vi "Teleop.vi"(10 "Match Info":T1={"Autonomous Elapsed Seconds"=0.0, "TeleOp Elapsed Seconds"=0.0, "Disabled Elapsed Seconds"=0.0, "Visited Autonomous"=FALSE, "Visited TeleOp"=FALSE, "Visited Disabled"=FALSE, "Autonomous Settings"={"Autonomous Style"=enum."Independent", "VI Refnum"=refnum}}, 11 "Call Context":T2) -> ()   [LabVIEW 2023]
doc: "This VI is called for each TeleOp packet received from the DS where the robot is not disabled. It is often used to read from the joysticks and update I/O or to update setpoints for timed control loops. It should complete and return within 20 milliseconds or it may miss DS packets."
uses:
  <vilib>/Rock Robotics/WPI/DriverStation/WPI_DriverStationDerivedRobotMode.ctl
  <vilib>/Rock Robotics/WPI/DriverStation/WPI_DriverStationMatch Info.ctl
  <vilib>/Rock Robotics/WPI/Utilities/WPI_GetSetVariantRefNum.vi
  <vilib>/Rock Robotics/Network Tables/NT Write Boolean Array.vi
  <vilib>/Rock Robotics/Network Tables/NT Write Numeric Array.vi
  <vilib>/Rock Robotics/Network Tables/NT Read Boolean.vi
  <vilib>/Rock Robotics/Network Tables/NT Read Number.vi
  <vilib>/Rock Robotics/WPI/ThirdParty/Phoenix-LabVIEW/Pigeon IMU/CTRE_PigeonIMU_GetYPR.vi
  <vilib>/Rock Robotics/Network Tables/NT Write Float.vi
panel:
  out "Yaw":dbl(knob) scale=-180.0..180.0
  out "Sample Slider 0":dbl(slide) scale=0.0..5.0
  out "Sample Boolean 1":bool
  out "Sample Boolean 0":bool
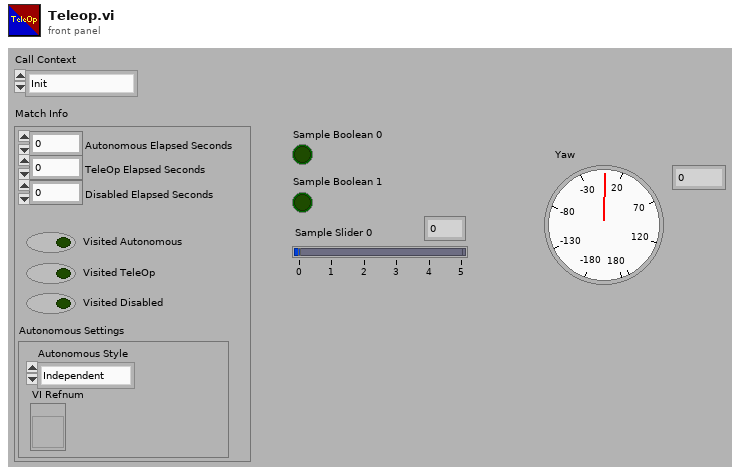
[diagram p1: front panel]
types:
  T1 = typedef "WPI_DriverStationMatch Info.ctl" = cluster{"Autonomous Elapsed Seconds":dbl, "TeleOp Elapsed Seconds":dbl, "Disabled Elapsed Seconds":dbl, "Visited Autonomous":bool, "Visited TeleOp":bool, "Visited Disabled":bool, "Autonomous Settings":cluster{"Autonomous Style":enum16{"Iterative", "Independent"}, "VI Refnum":refnum<vi>}}
  T2 = typedef "WPI_DriverStationDerivedRobotMode.ctl" = enum16{"Init", "Execute", "Stop"}
  T3 = typedef "WPI_JoystickDevRef.ctl" = cluster{"Device":T4}
  T4 = typedef "WPI_JoystickDeviceEnum.ctl" = enum16{"USB 0", "USB 1", "USB 2", "USB 3", "USB 4", "USB 5"}
  T5 = typedef "CTRE_PigeonIMU_DeviceRef.ctl" = cluster{"DeviceStatus":errorcluster, "Device Number":u8, "Type":T6, "Device ID":u32, "Handle":u64, "UsageFrame":u32, "Library Path":path}
  T6 = typedef "CTRE_PigeonIMU_ConnectionType.ctl" = u32
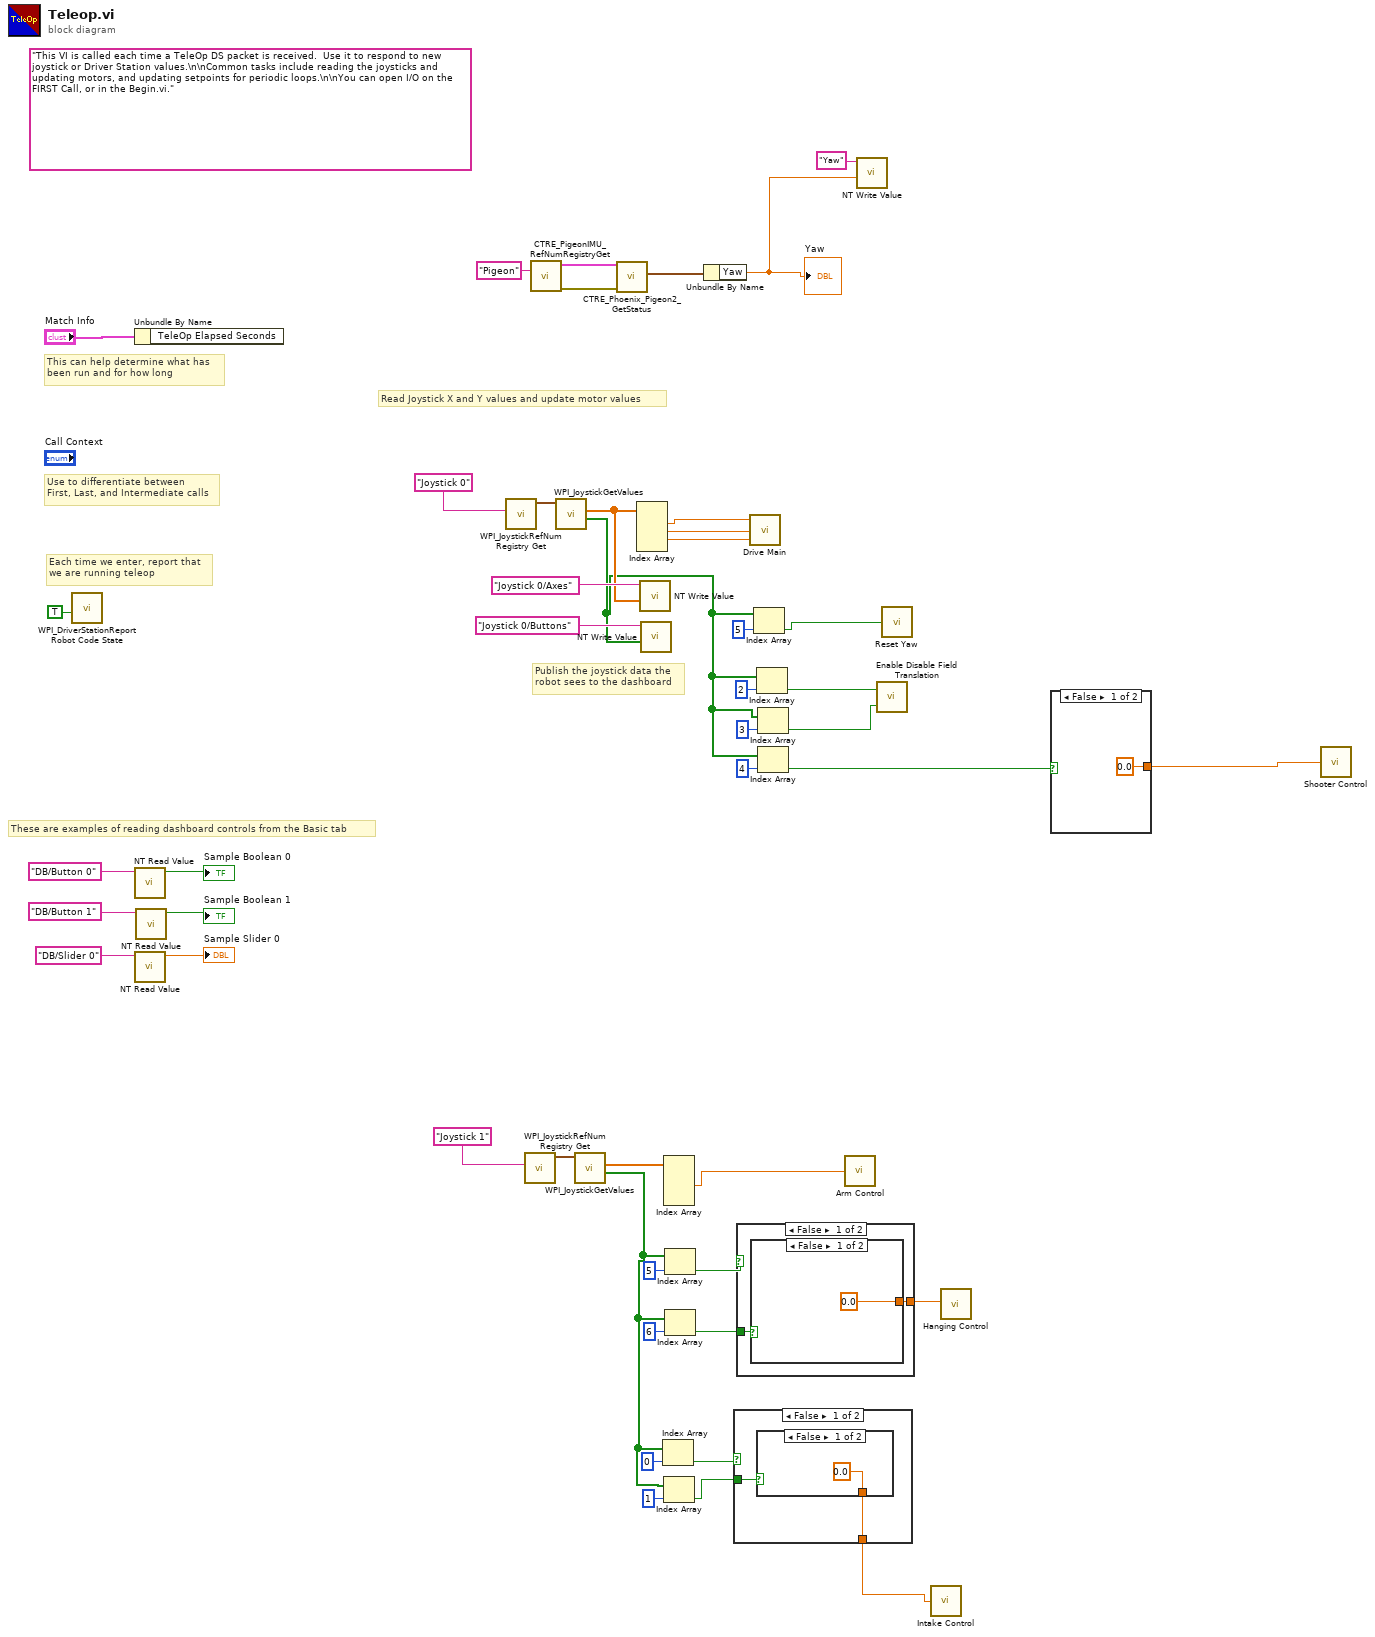
[diagram p0: block diagram]
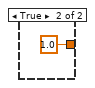
[diagram p2: hidden frame]
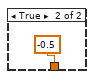
[diagram p3: hidden frame]
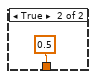
[diagram p4: hidden frame]
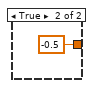
[diagram p5: hidden frame]
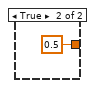
[diagram p6: hidden frame]
diagram:
  (unwired) "This VI is called each time a TeleOp DS packet is received.  Use it to respond to new joystick or Driver Station values.\n\nCommon tasks include reading the joysticks and updating motors, and updating setpoints for periodic loops.\n\nYou can open I/O on the FIRST Call, or in the Begin.vi."
  # "These are examples of reading dashboard controls from the Basic tab"
  # "Publish the joystick data the\nrobot sees to the dashboard"
  # "Each time we enter, report that\nwe are running teleop"
  # "Use to differentiate between\nFirst, Last, and Intermediate calls"
  # "This can help determine what has\nbeen run and for how long"
  # "Read Joystick X and Y values and update motor values"
  n1 = call <vilib>:"WPI_DriverStationReport Robot Code State.vi"("TeleOp"=TRUE ("Autonomous")) -> ()  [unwired: 10 in, 1 out]
  n2 = Unbundle By Name("Match Info") -> ()  [unwired: 1 out]
  n3 = call-poly <vilib>:"NT Read Value.vi"("name"="DB/Button 0" ("refnum name")) -> ("value"=→"Sample Boolean 0":bool)  [unwired: 8 in, 2 out]
  n4 = call-poly <vilib>:"NT Read Value.vi"("name"="DB/Slider 0" ("refnum name")) -> ("value"=→"Sample Slider 0":dbl)  [unwired: 8 in, 2 out]
  n5 = call-poly <vilib>:"NT Read Value.vi"("name"="DB/Button 1" ("refnum name")) -> ("value"=→"Sample Boolean 1":bool)  [unwired: 8 in, 2 out]
  n6 = call <vilib>:"WPI_JoystickRefNum Registry Get.vi"("refnum name"="Joystick 0") -> ("JoystickDevRef"=w45:T3)  [unwired: 1 in, 9 out]
  n7 = call <vilib>:"WPI_JoystickRefNum Registry Get.vi"("refnum name"="Joystick 1") -> ("JoystickDevRef"=w21:T3)  [unwired: 1 in, 9 out]
  n8 = call <vilib>:"CTRE_PigeonIMU_RefNumRegistryGet.vi"("refnum name"="Pigeon") -> ("error out"=w32:errorcluster, "PigeonIMUDevRef"=w33:T5)  [unwired: 9 in]
  n9 = call <vilib>:"WPI_JoystickGetValues.vi"("JoystickDevRef"=w45) -> ("Buttons"=w12:bool[], "Axes"=w41:dbl[])  [unwired: 6 in, 3 out]
  n10 = call <vilib>:"WPI_JoystickGetValues.vi"("JoystickDevRef"=w21) -> ("Buttons"=w8:bool[], "Axes"=w20:dbl[])  [unwired: 6 in, 3 out]
  n11 = call-poly <vilib>:"CTRE_Phoenix_Pigeon2_GetStatus.vi"("error in (no error)"=w32, "PigeonIMUDevRef"=w33) -> ("Yaw Pitch Roll"=w31:cluster{"Yaw":dbl, "Pitch":dbl, "Roll":dbl})  [unwired: 7 in, 2 out]
  n12 = Index Array(array=w41) -> (element #1=w5:dbl, element #2=w4:dbl, element #3=w3:dbl)  [unwired: 4 in, 1 out]
  n13 = call-poly <vilib>:"NT Write Value.vi"("value"=w41, "name"="Joystick 0/Axes" ("Name")) -> ()  [unwired: 9 in, 1 out]
  n14 = call-poly <vilib>:"NT Write Value.vi"("value"=w12, "name"="Joystick 0/Buttons" ("Name")) -> ()  [unwired: 9 in, 1 out]
  n15 = Index Array(array=w8, index=0) -> (element=w13:bool)
  n16 = Index Array(array=w20) -> (element #2=w6:dbl)  [unwired: 4 in, 3 out]
  n17 = Index Array(array=w8, index=1) -> (element=w7:bool)
  n18 = Index Array(array=w8, index=5) -> (element=w17:bool)
  n19 = Index Array(array=w8, index=6) -> (element=w16:bool)
  n20 = Unbundle By Name(w31) -> ("Yaw"=w29:dbl)
  "Yaw" <- w29
  n21 = case shown="False" w13 {
    tunnel: [w49 0.5 ("Output")] -> w1
    tunnel: w7 -> [w48 _]
    frame False {
      n22 = case shown="False" w48 {
        tunnel: [0.0 ("Output") -0.5 ("Output")] -> w49
        frame False {
        }
        frame True {
        }
      }
    }
    frame True {
    }
  }
  n23 = case shown="False" w17 {
    tunnel: w16 -> [w54 _]
    tunnel: [w53 0.5 ("Hanging Control")] -> w15
    frame False {
      n24 = case shown="False" w54 {
        tunnel: [0.0 ("Hanging Control") -0.5 ("Hanging Control")] -> w53
        frame False {
        }
        frame True {
        }
      }
    }
    frame True {
    }
  }
  n25 = call "Drive Main.vi"("spin"=w3, "In x"=w4, "In y"=w5) -> ()
  n26 = Index Array(array=w12, index=5) -> (element=w27:bool)
  n27 = Index Array(array=w12, index=2) -> (element=w24:bool)
  n28 = Index Array(array=w12, index=3) -> (element=w23:bool)
  n29 = Index Array(array=w12, index=4) -> (element=w10:bool)
  n30 = call "Arm Control.vi"("Arm Control"=w6) -> ()  [unwired: 1 out]
  n31 = call-poly <vilib>:"NT Write Value.vi"("value"=w29, "name"="Yaw") -> ()  [unwired: 9 in, 1 out]
  n32 = call "Enable Disable Field Translation.vi"("Disable"=w23, "Enable"=w24) -> ()  [unwired: 2 in]
  n33 = call "Reset Yaw.vi"("Reset"=w27) -> ()  [unwired: 1 in]
  n34 = call "Intake Control.vi"("Intake Setpoint"=w1) -> ()  [unwired: 1 in]
  n35 = call "Hanging Control.vi"("Hanging Control"=w15) -> ()  [unwired: 1 in]
  n36 = case shown="False" w10 {
    tunnel: [0.0 ("Output") 1.0 ("Output")] -> w2
    frame False {
    }
    frame True {
    }
  }
  n37 = call "Shooter Control.vi"("Setpoint"=w2) -> ()  [unwired: 1 in]
